vi "saveWaveform.vi"(0 "axe y label":string, 1 "axe x label":string, 2 "Waveform":waveform(dbl), 3 "x_zero":dbl, 4 "pt_off":dbl) -> ()   [LabVIEW 2013]
uses:
  <vilib>/Utility/file.llb/Write To Spreadsheet File (string).vi
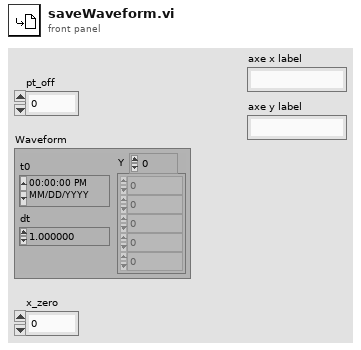
[diagram p1: front panel]
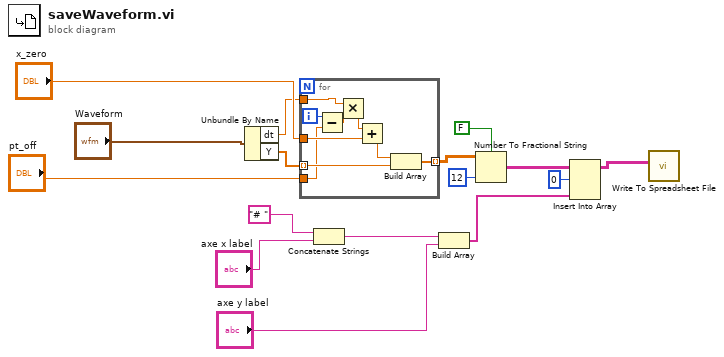
[diagram p0: block diagram]
diagram:
  n1 = Unbundle By Name("Waveform") -> ("dt"=w12:dbl, "Y"=w13:dbl[])
  n2 = for {
    tunnel: w12 -> [w25]
    tunnel: w13 -> [w22] mode=indexing
    tunnel: [w21] -> w11 mode=indexing
    tunnel: "x_zero" -> [w20]
    tunnel: "pt_off" -> [w17]
    i -> [w19]
    n3 = Subtract(x=w19, y=w17) -> (x-y=w18:dbl)
    n4 = Multiply(x=w25, y=w18) -> (x*y=w24:dbl)
    n5 = Add(x=w24, y=w20) -> (x+y=w23:dbl)
    n6 = Build Array(w23, w22) -> (w21:dbl[])
  }
  n7 = Concatenate Strings("# " ("string"), "axe x label") -> (w1:string)
  n8 = Build Array(w1, "axe y label") -> (w5:string[])
  n9 = Number To Fractional String(use system decimal point (T)=FALSE, number=w11, precision (6)=i16 12) -> (F-format string=w4:string[][])  [unwired: 1 in]
  n10 = Insert Into Array(array=w4, index (row)=0, new element=w5) -> (w6:string[][])  [unwired: 1 in]
  n11 = call-poly <vilib>:"Write To Spreadsheet File.vi"("2D data"=w6) -> ()  [unwired: 7 in, 1 out]
